vi "Agilent SNA Unflatten Driver Configuration.vi"(9 "SNA Configuration (\"\")":string) -> (1 "Configuration":T1={"BusType"=enum."GPIB", "GPIB Bus"=0, "GPIB Address"=16, "Pass Through Address"=19, "IP"=0, "SCIL Address"=16, "COM"=1, "Baud Rate"=enum."9600", "USB Device"=0, "Instrument S\\N"=""} {"USB Device" max=31 step=1}, 4 "Version":string)   [LabVIEW 2011]
uses:
  SNA Configuration.ctl
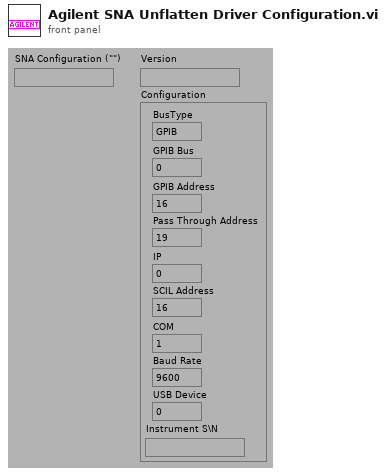
[diagram p1: front panel]
types:
  T1 = typedef "SNA Configuration.ctl" = cluster{"BusType":enum32{"GPIB", "LAN/IP", "Serial", "USB"}, "GPIB Bus":i32, "GPIB Address":i32, "Pass Through Address":i32, "IP":u32, "SCIL Address":i32, "COM":i32, "Baud Rate":enum32{"300", "600", "1200", "2400", "4800", "9600"}, "USB Device":i32, "Instrument S\\N":string}
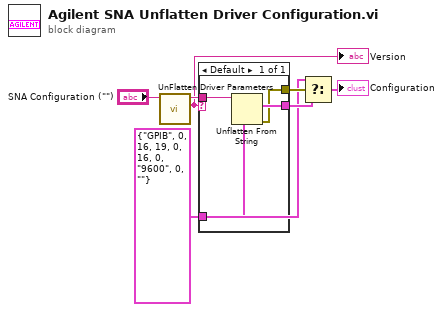
[diagram p0: block diagram]
diagram:
  w2 = T1 {"BusType"=enum."GPIB", "GPIB Bus"=0, "GPIB Address"=16, "Pass Through Address"=19, "IP"=0, "SCIL Address"=16, "COM"=0, "Baud Rate"=enum."9600", "USB Device"=0, "Instrument S\\N"=""} ("Configuration")
  n1 = call "UnFlatten Driver Parameters.vi"("Flattened Driver Parameters with Version (\"\")"="SNA Configuration (\"\")") -> ("Driver Version"=w1:string, "Flat Driver Parameters"=w3:string)  [unwired: 1 in, 4 out]
  "Version" <- w1
  n2 = case shown="Default" w1 {
    tunnel: [w11] -> w7
    tunnel: [w8] -> w5
    tunnel: w3 -> [w10]
    tunnel: w2 -> [w9]
    frame Default {
      n3 = Unflatten From String(type=w9, binary string=w10) -> (value=w11:T1, error out=w8:errorcluster)  [unwired: 1 in, 3 out]
    }
  }
  n4 = Select(t=w2, s=w5, f=w7) -> (s? t:f=→"Configuration":T1)
